vi "ReadWrite All Data.vi"(6 "Iteration":i32, 7 "Mode":T1, 8 "error in (no error)":errorcluster, 10 "ScheduledSDI":bool, 11 "RT Data in":T2 {"Label Transfer Config"."Block Data Refs"."Data Reference" format="%.0x"; "Status Config"."HWOut Dur Ref" format="%.0x"; "Status Config"."HWIn Dur Ref" format="%.0x"; "Status Config"."HWOut Count Ref" format="%.0x"; "Status Config"."HWIn Count Ref" format="%.0x"; "Status Config"."Error Data Ref" format="%.0x"; "HWOutput Channels"."Labels Settings"."Driver Data"."Num Bits" min=1 max=32; "HWOutput Channels"."Labels Settings"."Driver Data"."Start Bit" min=8 max=31; "HWOutput Channels"."Labels Settings"."Block Data Refs"."Data Reference" format="%.0x"; "HWOutput Channels"."Labels Settings"."Label" format="%.0o"; "HWInput Channels"."Labels Settings"."Driver Data"."Num Bits" min=1 max=32; "HWInput Channels"."Labels Settings"."Driver Data"."Start Bit" min=8 max=31; "HWInput Channels"."Labels Settings"."Block Data Refs"."Data Reference" format="%.0x"; "HWInput Channels"."Labels Settings"."Label" format="%.0o"}) -> (0 "error out":errorcluster, 3 "RT Data out":T2 {"Label Transfer Config"."Block Data Refs"."Data Reference" format="%.0x"; "Status Config"."HWOut Dur Ref" format="%.0x"; "Status Config"."HWIn Dur Ref" format="%.0x"; "Status Config"."HWOut Count Ref" format="%.0x"; "Status Config"."HWIn Count Ref" format="%.0x"; "Status Config"."Error Data Ref" format="%.0x"; "HWOutput Channels"."Labels Settings"."Driver Data"."Num Bits" min=1 max=32; "HWOutput Channels"."Labels Settings"."Driver Data"."Start Bit" min=8 max=31; "HWOutput Channels"."Labels Settings"."Block Data Refs"."Data Reference" format="%.0x"; "HWOutput Channels"."Labels Settings"."Label" format="%.0o"; "HWInput Channels"."Labels Settings"."Driver Data"."Num Bits" min=1 max=32; "HWInput Channels"."Labels Settings"."Driver Data"."Start Bit" min=8 max=31; "HWInput Channels"."Labels Settings"."Block Data Refs"."Data Reference" format="%.0x"; "HWInput Channels"."Labels Settings"."Label" format="%.0o"})   [LabVIEW 2011, in "AIT 1553 Custom Device.lvlib"]
uses:
  AIT 1553 Custom Device.lvlib
  RT Controls/RT Data.ctl
  RT Controls/RT HW Channel.ctl
  RT Controls/RT Label Settings.ctl
  Controls and Global/Label.ctl
  Controls and Global/transferPeriod.ctl
  <vilib>/NI Veristand/Custom Device API/Block Data Reference.ctl
  <vilib>/NI Veristand/Custom Device API/Data Reference.ctl
  RT Controls/Driver Data.ctl
  Controls and Global/Start Bit.ctl
  Controls and Global/Number of Bits.ctl
  RT Controls/Error Qs.ctl
  RT Controls/Status Channels Config.ctl
  RT Controls/FIFO.ctl
  RT Controls/Label Transfer Config.ctl
  <userlib>/ARINC-429/vi/enum/Owl429HardwareSource.ctl
  RT Controls/ReadWrite Selector.ctl
  Search Label Array for Index of Label.vi
  ReadWrite Label.vi
  Calculate Buffer Index for Label Data (AIM_AIT).vi
  Calculate Number of Labels Available to Read (AIM_AIT).vi
  <vilib>/NI Veristand/Custom Device API/NI VeriStand - Set Channel Values by Block Data Reference.vi
  Write outgoing label data.vi
  <vilib>/NI Veristand/Custom Device API/NI VeriStand - Get Channel Values by Block Data Reference.vi
  Read incoming label data.vi
  Double to selected bits.vi
  SubVIs/Word to double.vi
  <userlib>/ARINC-429/vi/IRxChronMonChannel/Owl429_IRxChronMonChannel_read.vi
  <instrlib>/AIT 429/Public/Utility/AIT 429 Get SDI.vi
  <instrlib>/AIT 429/Public/Utility/AIT 429 Get Label.vi
  <vilib>/NI Veristand/Custom Device API/Global Data Refs.vi
  <instrlib>/AIT 429/Public/Tx/Data/AIT 429 Set Scheduled Label Datum.vi
  <instrlib>/AIT 429/Public/Tx/Data/AIT 429 Get Scheduled Label Datum.vi
  <vilib>/NI Veristand/Custom Device API/Custom Device API.lvlib
  <userlib>/ARINC-429/Owl429.lvlib
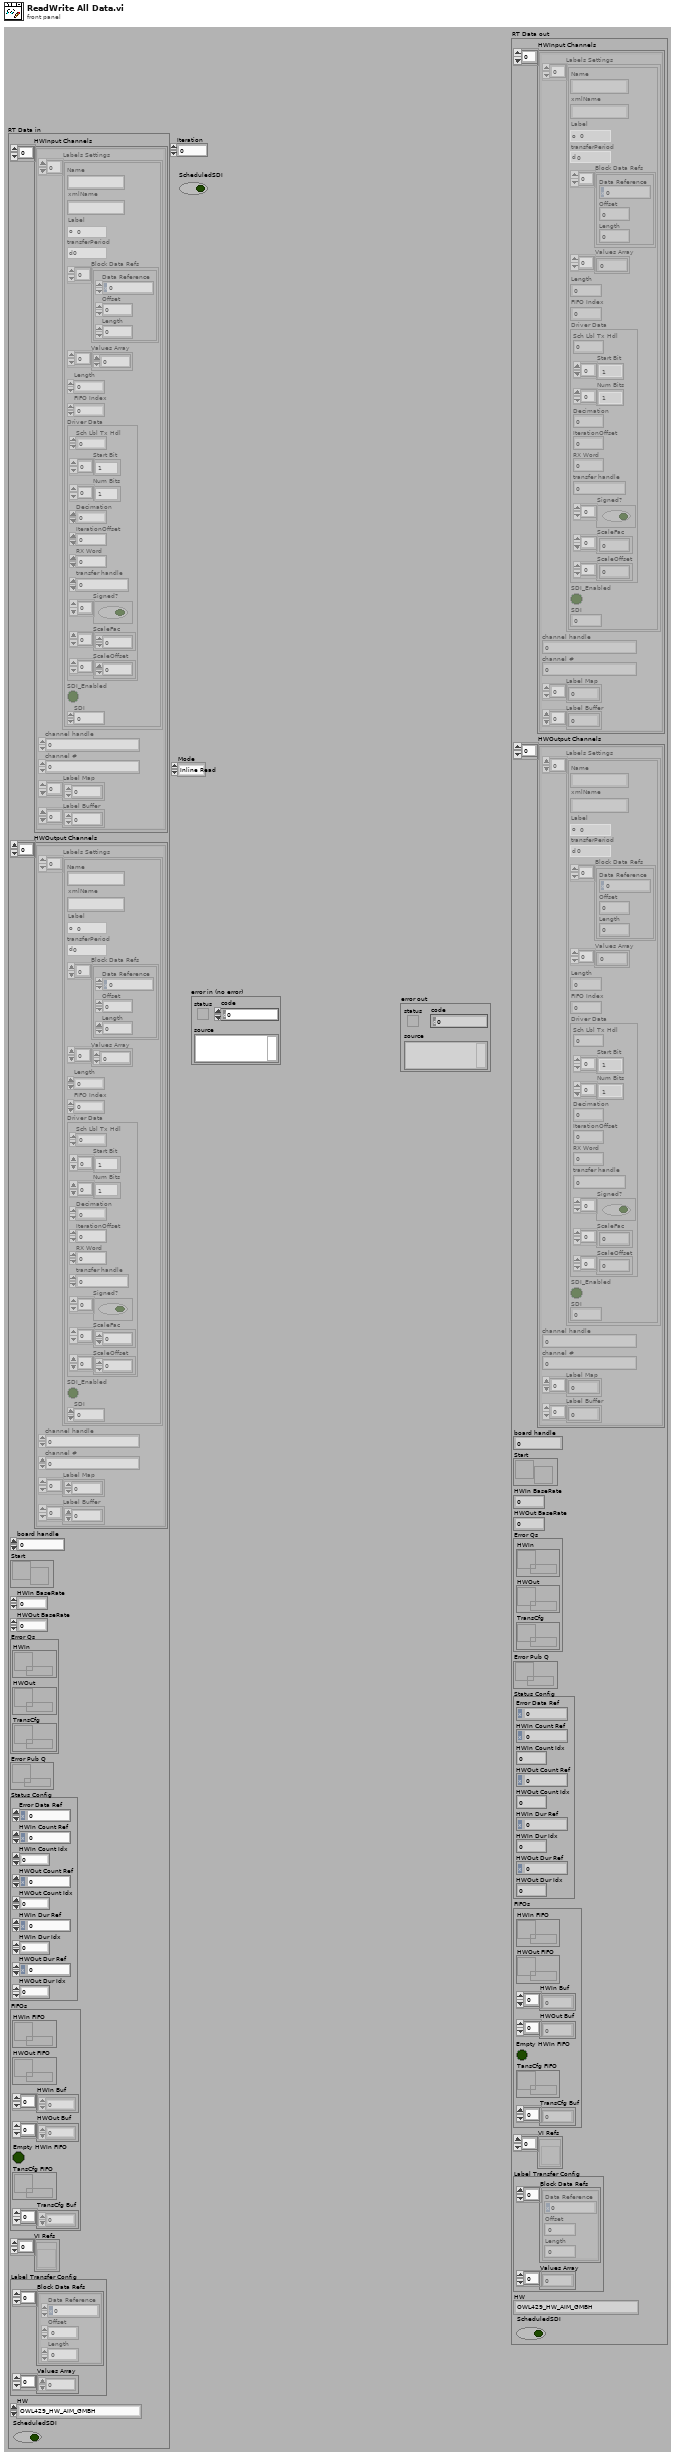
[diagram p1: front panel]
types:
  T1 = typedef "AIT 1553 Custom Device.lvlib/ReadWrite Selector.ctl" = enum16{"Inline Read", "Inline Write", "Async HWIn", "Async HWOut"}
  T2 = typedef "AIT 1553 Custom Device.lvlib/RT Data.ctl" = cluster{"HWInput Channels":T3[], "HWOutput Channels":T3[], "board handle":u32, "Start":refnum<notifier>, "HWIn BaseRate":i64, "HWOut BaseRate":i64, "Error Qs":T12, "Error Pub Q":refnum<queue>, "Status Config":T13, "FIFOs":T14, "VI Refs":refnum<vi>[], "Label Transfer Config":T15, "HW":T16, "ScheduledSDI":bool}
  T3 = typedef "AIT 1553 Custom Device.lvlib/RT HW Channel.ctl" = cluster{"Labels Settings":T4[], "channel handle":u32, "channel #":u16, "Label Map":i32[], "Label Buffer":u32[]}
  T4 = typedef "AIT 1553 Custom Device.lvlib/RT Label Settings.ctl" = cluster{"Name":string, "xmlName":string, "Label":T5, "transferPeriod":T6, "Block Data Refs":T7[], "Values Array":dbl[], "Length":i32, "FIFO Index":i32, "Driver Data":T9, "SDI_Enabled":bool, "SDI":u8}
  T5 = typedef "AIT 1553 Custom Device.lvlib/Label.ctl" = u8
  T6 = typedef "AIT 1553 Custom Device.lvlib/transferPeriod.ctl" = u32
  T7 = typedef "Custom Device API.lvlib/Block Data Reference.ctl" = cluster{"Data Reference":T8, "Offset":i32, "Length":i32}
  T8 = typedef "Custom Device API.lvlib/Data Reference.ctl" = i32
  T9 = typedef "AIT 1553 Custom Device.lvlib/Driver Data.ctl" = cluster{"Sch Lbl Tx Hdl":u32, "Start Bit":T10[], "Num Bits":T11[], "Decimation":i32, "IterationOffset":i32, "RX Word":u32, "transfer handle":u32, "Signed?":bool[], "ScaleFac":dbl[], "ScaleOffset":dbl[]}
  T10 = typedef "AIT 1553 Custom Device.lvlib/Start Bit.ctl" = i32
  T11 = typedef "AIT 1553 Custom Device.lvlib/Number of Bits.ctl" = i32
  T12 = typedef "AIT 1553 Custom Device.lvlib/Error Qs.ctl" = cluster{"HWIn":refnum<queue>, "HWOut":refnum<queue>, "TransCfg":refnum<queue>}
  T13 = typedef "AIT 1553 Custom Device.lvlib/Status Channels Config.ctl" = cluster{"Error Data Ref":T8, "HWIn Count Ref":T8, "HWIn Count Idx":i32, "HWOut Count Ref":T8, "HWOut Count Idx":i32, "HWIn Dur Ref":T8, "HWIn Dur Idx":i32, "HWOut Dur Ref":T8, "HWOut Dur Idx":i32}
  T14 = typedef "AIT 1553 Custom Device.lvlib/FIFO.ctl" = cluster{"HWIn FIFO":refnum<k33>, "HWOut FIFO":refnum<k33>, "HWIn Buf":dbl[], "HWOut Buf":dbl[], "Empty HWIn FIFO":bool, "TansCfg FIFO":refnum<k33>, "TransCfg Buf":dbl[]}
  T15 = typedef "AIT 1553 Custom Device.lvlib/Label Transfer Config.ctl" = cluster{"Block Data Refs":T7[], "Values Array":dbl[]}
  T16 = typedef "Owl429.lvlib/Owl429HardwareSource.ctl" = enum16{"OWL429_HW_AIM_GMBH", "OWL429_HW_AIT"}
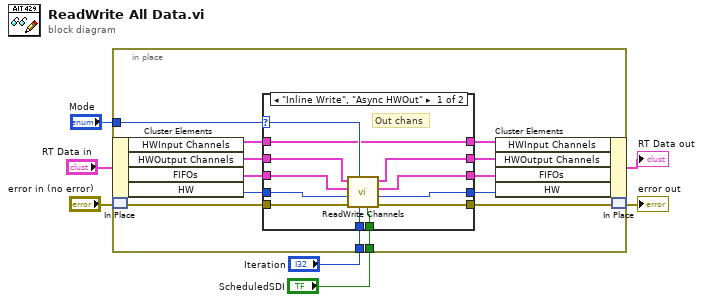
[diagram p0: block diagram]
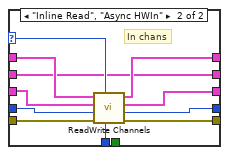
[diagram p2: hidden frame]
diagram:
  n1 = in-place {
    in-place-border: "Mode" -> [w14]
    in-place-border: "Iteration" -> [w11]
    in-place-border: "ScheduledSDI" -> [w8]
    n2 = in-place-cluster #1("RT Data in") -> ("HWInput Channels"=w20:T3[], "HWOutput Channels"=w13:T3[], "FIFOs"=w16:T14, "HW"=w10:T16)
    n3 = in-place-match #2("error in (no error)") -> (w18:errorcluster)
    n4 = case shown="\"Inline Write\", \"Async HWOut\"" w14 {
      selector: w14 -> [w31 w39]
      tunnel: w20 -> [w27 w43]
      tunnel: [w27 w42] -> w19
      tunnel: w18 -> [w32 w41]
      tunnel: [w30 w40] -> w17
      tunnel: w16 -> [w24 w36]
      tunnel: [w25 w35] -> w15
      tunnel: w13 -> [w29 w38]
      tunnel: [w28 w38] -> w12
      tunnel: w11 -> [w26 w37]
      tunnel: w10 -> [w23 w34]
      tunnel: [w22 w33] -> w9
      tunnel: w8 -> [w21 _]
      frame "Inline Write", "Async HWOut" {
        # "Out chans"
        n5 = call "ReadWrite Channels.vi"("ScheduledSDI"=w21, "Iteration"=w26, "Mode"=w31, "error in (no error)"=w32, "hardware  in"=w23, "FIFOs In"=w24, "Channels In"=w29) -> ("error out"=w30:errorcluster, "hardware  out"=w22:T16, "FIFOs Out"=w25:T14, "Channels Out"=w28:T3[])  [unwired: 1 in]
      }
      frame "Inline Read", "Async HWIn" {
        # "In chans"
        n6 = call "ReadWrite Channels.vi"("Iteration"=w37, "Mode"=w39, "error in (no error)"=w41, "hardware  in"=w34, "FIFOs In"=w36, "Channels In"=w43) -> ("error out"=w40:errorcluster, "hardware  out"=w33:T16, "FIFOs Out"=w35:T14, "Channels Out"=w42:T3[])  [unwired: 2 in]
      }
    }
    n7 = in-place-cluster #1("HWInput Channels"=w19, "HWOutput Channels"=w12, "FIFOs"=w15, "HW"=w9) -> (→"RT Data out":T2)
    n8 = in-place-match #2(w17) -> (→"error out":errorcluster)
  }
